vi "oa_Convert Pulse Positions to Speed (No State).vi"(6 "state in":T1, 7 "reset?":bool, 9 "waveform duration":dbl, 11 "speed position info":T2) -> (3 "speed [RPM]":dbl, 4 "state out":T1)   [LabVIEW 2017]
uses:
  <vilib>/addons/Sound and Vibration/Order Analysis/Misc/OAT Position Info.ctl
  <vilib>/addons/_NISVFA/_Shared subVIs/Common/svc_Get Array Subset (Index).vi
  <vilib>/addons/_NISVFA/_Shared subVIs/Common/svc_Coerce Index and Length.vi
  <vilib>/addons/_NISVFA/_Shared subVIs/Common/svc_Conditional Merge Error.vi
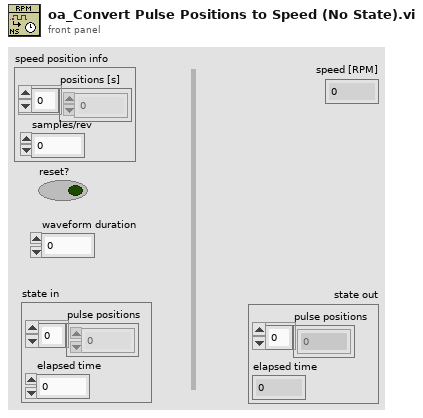
[diagram p1: front panel]
types:
  T1 = cluster{"pulse positions":dbl[], "elapsed time":dbl}
  T2 = typedef "OAT Position Info.ctl" = cluster{"positions [s]":dbl[], "samples/rev":dbl}
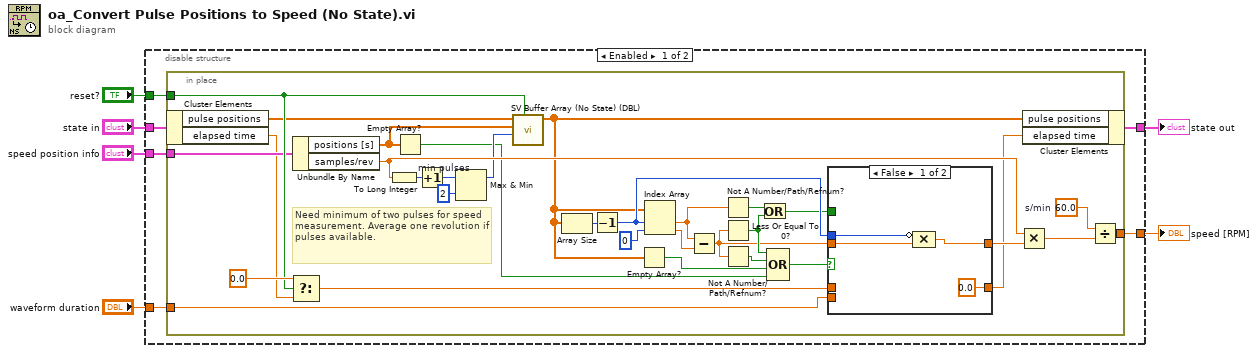
[diagram p0: block diagram]
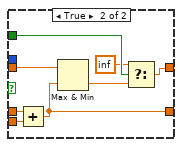
[diagram p2: hidden frame]
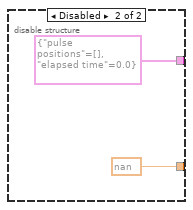
[diagram p3: hidden frame]
diagram:
  n1 = disable-structure shown="Enabled" {
    disable-tunnel: "reset?" -> [w12 _]
    disable-tunnel: "waveform duration" -> [w11 _]
    disable-tunnel: "speed position info" -> [w10 _]
    disable-tunnel: [w9 nan] -> w3
    disable-tunnel: "state in" -> [w8 _]
    disable-tunnel: [w7 T1 {"pulse positions"=[], "elapsed time"=0.0} ("state in")] -> w1
    frame Enabled {
      n2 = in-place {
        in-place-border: w12 -> [w42]
        in-place-border: w11 -> [w41]
        in-place-border: w10 -> [w32]
        in-place-border: [w25] -> w9
        w36 = 2  # min pulses
        w23 = 60.0  # s/min
        # "Need minimum of two pulses for speed measurement. Average one revolution if pulses available."
        n3 = in-place-cluster #1(w8) -> ("pulse positions"=w16:dbl[], "elapsed time"=w15:dbl)
        n4 = Select(t=0.0, s=w42, f=w15) -> (s? t:f=w43:dbl)
        n5 = Unbundle By Name(w32) -> ("positions [s]"=w33:dbl[], "samples/rev"=w40:dbl)
        n6 = To Long Integer(number=w40) -> (32bit integer=w34:i32)
        n7 = Empty Array?(array=w33) -> (empty?=w22:bool)
        n8 = Increment(x=w34) -> (x+1=w38:i32)
        n9 = Max & Min(x=w38, y=w36) -> (max(x,y)=w35:i32)  [unwired: 1 out]
        n10 = call <vilib>:"SV Buffer Array (No State) (DBL).vi"("clear buffer (False)"=w42, "buffer length  [samples] (-1 = unlimited)"=w35, "Y"=w33, "buffer in"=w16) -> ("buffer out"=w14:dbl[])  [unwired: 7 in]
        n11 = Array Size(array=w14) -> (size(s)=w37:i32)
        n12 = Decrement(x=w37) -> (x-1=w39:i32)
        n13 = Empty Array?(array=w14) -> (empty?=w26:bool)
        n14 = Index Array(array=w14, index #1=w39, index #2=0 ("index")) -> (element #1=w17:dbl, element #2=w30:dbl)
        n15 = Subtract(x=w17, y=w30) -> (x-y=w29:dbl)
        n16 = Not A Number/Path/Refnum?(number/path/refnum=w17) -> (NaN/Path/Refnum?=w27:bool)
        n17 = Less Or Equal To 0?(x=w29) -> (x <= 0?=w31:bool)
        n18 = Not A Number/Path/Refnum?(number/path/refnum=w29) -> (NaN/Path/Refnum?=w20:bool)
        n19 = Or(x=w27, y=w31) -> (x .or. y?=w28:bool)
        n20 = Compound Arithmetic op=OR(w31, w20, w26, w22) -> (w21:bool)
        n21 = case shown="False" w21 {
          tunnel: [w45 w54] -> w18
          tunnel: w29 -> [w46 w50]
          tunnel: w28 -> [_ w56]
          tunnel: w41 -> [_ w53]
          tunnel: w43 -> [_ w52]
          tunnel: [0.0 w51] -> w13
          tunnel: w39 -> [w47 _]
          frame False {
            n22 = Compound Arithmetic op=MULTIPLY(invert w47, w46) -> (w45:dbl)
          }
          frame True {
            n23 = Add(x=w52, y=w53) -> (x+y=w51:dbl)
            n24 = Max & Min(x=w50, y=w51) -> (min(x,y)=w49:dbl)  [unwired: 1 out]
            n25 = Select(t=inf, s=w56, f=w49) -> (s? t:f=w54:dbl)
          }
        }
        n26 = Multiply(x=w40, y=w18) -> (x*y=w24:dbl)
        n27 = in-place-cluster #1("pulse positions"=w14, "elapsed time"=w13) -> (w7:T1)
        n28 = Divide(x=w23, y=w24) -> (x/y=w25:dbl)
      }
    }
    frame Disabled {
    }
  }
  "speed [RPM]" <- w3
  "state out" <- w1
